vi "New Project.vi"(9 "DBSet":T1={"Server"="172.20.23.107", "DB"="HTPSDB", "PSW"="data'songyy", "User"="sa"}, 10 "UserID":string="L043460", 11 "厂区":string="清溪") -> ()   [LabVIEW 2011] (continued)
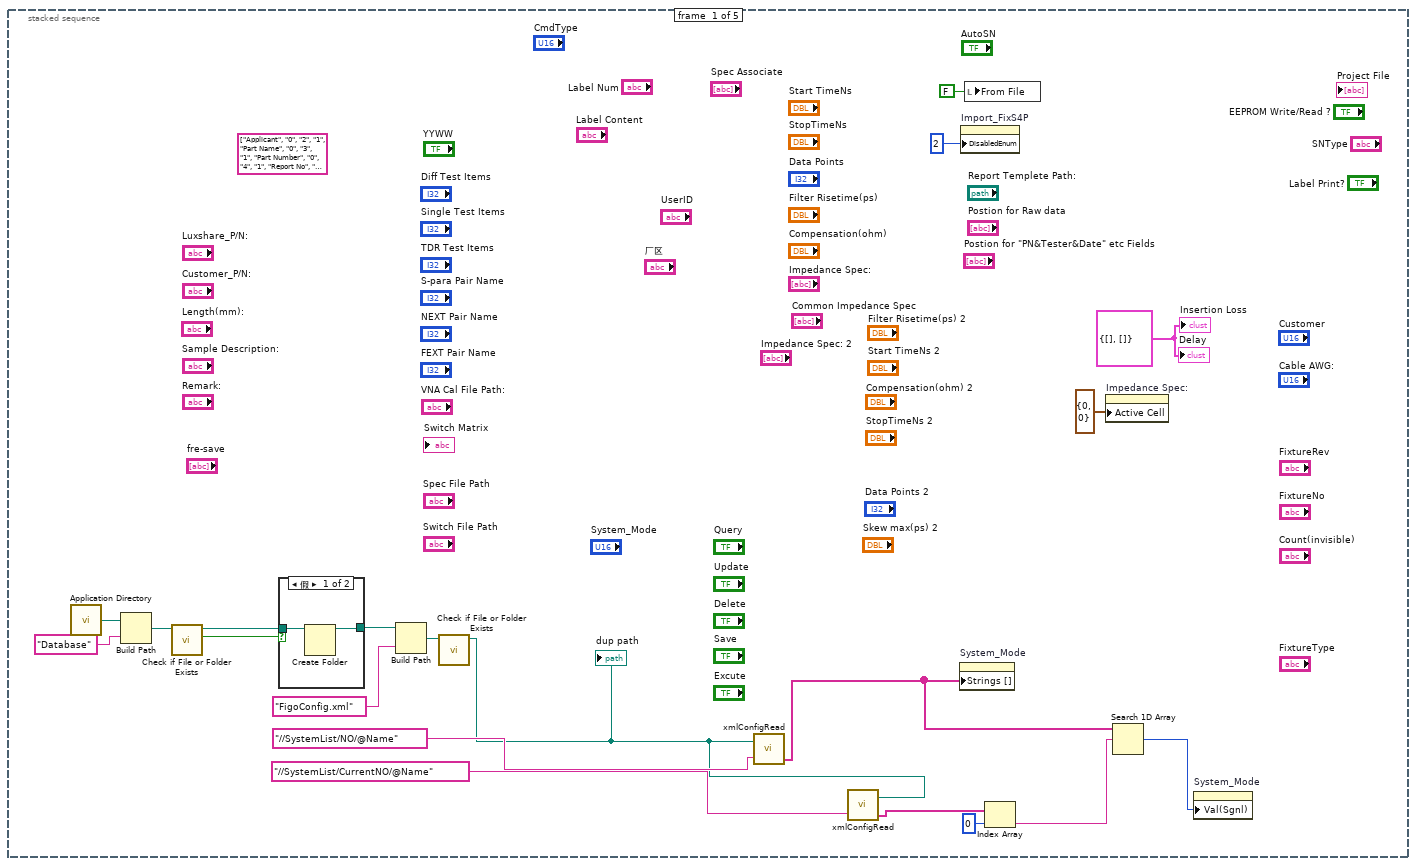
[diagram p3: hidden frame]
                          }
                          frame True {
                            n930 = local read "Luxshare_P/N:"() -> (w1140:string)
                            n931 = local read "Project File"() -> (w1139:string[])
                            n932 = local read "Local"() -> (w1138:bool)
                            n933 = case shown="真" w1138 {
                              tunnel: w1139 -> [w1145 w1157]
                              tunnel: w1140 -> [_ w1165]
                              tunnel: w1137 -> [w1141 _]
                              frame False {
                                (unwired) string[] ["LuxsharePN", "CustomerPN", "Customer", "Prjinf", "SampleDes", "AWG", "Length", "Spec", "SwitchMatrix", "EEPROMTF", "FixtureNo", "LabelTF", "LabelNum", "LabelC", "Remark", "AutoSN", "FrePoints"] ("列名")
                                # "保存至数据库"
                                n934 = call "sql-writeinfo_vproject.vi"("操作模式"=enum16{"写入数据", "更改数据"}."写入数据", "列名"=string[] ["LuxsharePN", "CustomerPN", "Customer", "Prjinf", "SampleDes", "AWG", "Length", "Spec", "SwitchMatrix", "EEPROMTF", "FixtureNo", "LabelTF", "LabelNum", "LabelC", "Remark", "AutoSN", "FrePoints", "Switch_File_Path", "Spec_File_Path", "Spec_Points", "HardWare_Mode", "Factory", "LastLog"], "DBSet"=w1141, "值"=w1145) -> ("简单报错"=w1143:string, "status"=w1144:bool)  [unwired: 14 in]
                                n935 = case shown="假" w1144 {
                                tunnel: w1143 -> [_ w1156]
                                frame False {
                                # "清空操作"
                                n936 = control-ref of="Spec Associate"() -> (w1147:refnum<vi>)
                                n937 = control-ref of="Report Templete Path:"() -> (w1150:refnum<vi>)
                                n938 = control-ref of="Data Points"() -> (w1149:refnum<vi>)
                                n939 = local read "bool"() -> (w1148:refnum<vi>[])
                                n940 = One Button Dialog(message="Save Finished!" ("消息")) -> ()  [unwired: 1 in, 1 out]
                                n941 = local read "number"() -> (w1151:refnum<vi>[])
                                n942 = local read "string"() -> (w1154:refnum<vi>[])
                                n943 = local read "chart"() -> (w1152:refnum<vi>[])
                                n944 = local read "list"() -> (w1153:refnum<vi>[])
                                n945 = call "_wmg_initAllCtrls.vi"("chart"=w1152, "number"=w1151, "list"=w1153, "string"=w1154, "bool"=w1148, "Spec _Data"=w1147, "Data Points"=w1149, "Report Templete Path:"=w1150) -> ()
                                }
                                frame True {
                                n946 = One Button Dialog(message=w1156) -> ()  [unwired: 1 in, 1 out]
                                }
                                }
                              }
                              frame True {
                                n947 = call <vilib>:"Application Directory.vi"() -> ("Application Directory"=w1164:path)
                                n948 = Concatenate Strings("Database\\" ("字符串"), w1165, ".hpj" ("字符串")) -> (w1163:string)
                                n949 = Build Path(base path=w1164, name or relative path=w1163) -> (appended path=w1160:path)
                                n950 = call <vilib>:"Check if File or Folder Exists.vi"("path"=w1160) -> ("file or folder exists?"=w1159:bool, "dup path"=w1158:path)  [unwired: 8 in, 1 out]
                                n951 = case shown="真" w1159 {
                                tunnel: w1158 -> [w1169 w1179]
                                tunnel: w1157 -> [w1168 w1178]
                                frame False {
                                # "清空操作"
                                n952 = control-ref of="Spec Associate"() -> (w1166:refnum<vi>)
                                n953 = One Button Dialog(message="Local file save Finished!" ("消息")) -> ()  [unwired: 1 in, 1 out]
                                n954 = control-ref of="Report Templete Path:"() -> (w1175:refnum<vi>)
                                n955 = control-ref of="Data Points"() -> (w1176:refnum<vi>)
                                n956 = local read "bool"() -> (w1167:refnum<vi>[])
                                n957 = Write to Binary File(file (use dialog)=w1169, data=w1168, 9:T8."big-endian, network order" ("字节顺序(0:big-endian, network order)")) -> ()  [unwired: 3 in, 3 out]
                                n958 = local read "number"() -> (w1174:refnum<vi>[])
                                n959 = local read "string"() -> (w1171:refnum<vi>[])
                                n960 = local read "chart"() -> (w1173:refnum<vi>[])
                                n961 = local read "list"() -> (w1172:refnum<vi>[])
                                n962 = call "_wmg_initAllCtrls.vi"("chart"=w1173, "number"=w1174, "list"=w1172, "string"=w1171, "bool"=w1167, "Spec _Data"=w1166, "Data Points"=w1176, "Report Templete Path:"=w1175) -> ()
                                }
                                frame True {
                                n963 = Two Button Dialog(message="该PN的文件已经存在\n是否覆盖？", 1:"取消" ("F按钮名称（“取消”）"), 2:"覆盖" ("T按钮名称（“确定”）")) -> (T button?=w1180:bool)
                                n964 = case shown="真" w1180 {
                                tunnel: w1179 -> [_ w1185]
                                tunnel: w1178 -> [_ w1184]
                                frame False {
                                }
                                frame True {
                                n965 = stacked-sequence {
                                tunnel: w1185 -> [w1188 _]
                                tunnel: w1184 -> [w1186 _]
                                frame #0 {
                                n966 = One Button Dialog(message="Coved successfully!" ("消息")) -> ()  [unwired: 1 in, 1 out]
                                n967 = Write to Binary File(file (use dialog)=w1188, data=w1186, 9:T8."big-endian, network order" ("字节顺序(0:big-endian, network order)")) -> ()  [unwired: 3 in, 3 out]
                                }
                                frame #1 {
                                # "清空操作"
                                n968 = control-ref of="Report Templete Path:"() -> (w1195:refnum<vi>)
                                n969 = control-ref of="Data Points"() -> (w1196:refnum<vi>)
                                n970 = control-ref of="Spec Associate"() -> (w1190:refnum<vi>)
                                n971 = local read "number"() -> (w1194:refnum<vi>[])
                                n972 = local read "string"() -> (w1191:refnum<vi>[])
                                n973 = local read "chart"() -> (w1193:refnum<vi>[])
                                n974 = local read "list"() -> (w1192:refnum<vi>[])
                                n975 = call "_wmg_initAllCtrls.vi"("chart"=w1193, "number"=w1194, "list"=w1192, "string"=w1191, "Spec _Data"=w1190, "Data Points"=w1196, "Report Templete Path:"=w1195) -> ()  [unwired: 1 in]
                                }
                                }
                                }
                                }
                                }
                                }
                              }
                            }
                          }
                        }
                      }
                      frame #5 {
                        n976 = property on="Update" class="Bool (严格)"("DisabledEnum"=T5."Disabled and Grayed Out" ("禁用")) -> ()  [unwired: 2 in, 2 out]
                        n977 = property on="Delete" class="Bool (严格)"("DisabledEnum"=T5."Disabled and Grayed Out" ("禁用")) -> ()  [unwired: 2 in, 2 out]
                        n978 = property on="Luxshare_P/N:" class="Str"("DisabledEnum"=T5."Disabled and Grayed Out" ("禁用")) -> ()  [unwired: 2 in, 2 out]
                        n979 = local write "Query"(FALSE ("Query")) -> ()
                        n980 = local write "Update"(FALSE ("Query")) -> ()
                        n981 = local write "Delete"(FALSE ("Query")) -> ()
                        n982 = local write "Save"(FALSE ("Query")) -> ()
                      }
                    }
                  }
                  frame #2 {
                    w1205 = u16 0 items=["", "Common", "H3C psw 10G", "H3C psw 28G"] ("CmdType")
                    # "清空数组"
                    n983 = control-ref of="Spec Associate"() -> (w1204:refnum<vi>)
                    n984 = control-ref of="Report Templete Path:"() -> (w1208:refnum<vi>)
                    n985 = control-ref of="Data Points"() -> (w1207:refnum<vi>)
                    n986 = local write "CmdType"(w1205) -> ()
                    n987 = local read "bool"() -> (w1206:refnum<vi>[])
                    n988 = local read "number"() -> (w1209:refnum<vi>[])
                    n989 = local read "string"() -> (w1212:refnum<vi>[])
                    n990 = local read "chart"() -> (w1210:refnum<vi>[])
                    n991 = local read "list"() -> (w1211:refnum<vi>[])
                    n992 = call "_wmg_initAllCtrls.vi"("chart"=w1210, "number"=w1209, "list"=w1211, "string"=w1212, "bool"=w1206, "Spec _Data"=w1204, "Data Points"=w1207, "Report Templete Path:"=w1208) -> ()
                    n993 = property on="Update" class="Bool (严格)"("DisabledEnum"=T5."Disabled and Grayed Out" ("禁用")) -> ()  [unwired: 2 in, 2 out]
                    n994 = property on="Delete" class="Bool (严格)"("DisabledEnum"=T5."Disabled and Grayed Out" ("禁用")) -> ()  [unwired: 2 in, 2 out]
                    n995 = property on="Luxshare_P/N:" class="Str"("DisabledEnum"=T5."Disabled and Grayed Out" ("禁用")) -> ()  [unwired: 2 in, 2 out]
                    n996 = local write "Query"(FALSE ("Query")) -> ()
                    n997 = local write "Update"(FALSE ("Query")) -> ()
                    n998 = local write "Delete"(FALSE ("Query")) -> ()
                    n999 = local write "Save"(FALSE ("Query")) -> ()
                  }
                }
              }
              frame 10 {
                # "delete"
                n1000 = stacked-sequence {
                  tunnel: w1220 -> [w1221 _]
                  frame #0 {
                    n1001 = local read "Local"() -> (w1222:bool)
                    n1002 = case shown="假" w1222 {
                      tunnel: w1221 -> [w1223 _]
                      frame False {
                        n1003 = local read "Luxshare_P/N:"() -> (w1232:string)
                        n1004 = property on="System_Mode" class="Ring (严格)"() -> ("RingText.Text"=w1228:string)  [unwired: 2 in, 2 out]
                        n1005 = local read "厂区"() -> (w1224:string)
                        n1006 = call "_wmg_HardModetoHardModewhereConnect.vi"("Input"=w1228, "Factory"=w1224) -> ("Output"=w1226:string)
                        n1007 = call "_wmg_PNtoPNwhereConnect.vi"("Input"=w1232) -> ("Output"=w1227:string)
                        n1008 = Concatenate Strings(w1227, w1226) -> (w1225:string)
                        n1009 = call "sql-delete.vi"("操作模式"=T9."删除数据", "DBSet"=w1223, "限定条件"=w1225) -> ("错误类型"=w1229:string, "status"=w1230:bool)  [unwired: 15 in]
                        n1010 = case shown="假" w1230 {
                          tunnel: ["数据删除成功！" ("消息") w1235] -> w1231
                          tunnel: w1229 -> [_ w1235]
                          frame False {
                          }
                          frame True {
                          }
                        }
                        n1011 = One Button Dialog(message=w1231) -> ()  [unwired: 1 in, 1 out]
                      }
                      frame True {
                        n1012 = local read "Luxshare_P/N:"() -> (w1241:string)
                        n1013 = call <vilib>:"Application Directory.vi"() -> ("Application Directory"=w1245:path)
                        n1014 = Concatenate Strings("Database\\" ("字符串"), w1241, ".hpj" ("字符串")) -> (w1244:string)
                        n1015 = Build Path(base path=w1245, name or relative path=w1244) -> (appended path=w1240:path)
                        n1016 = Delete(path (use dialog)=w1240) -> (error out=w1236:errorcluster)  [unwired: 4 in, 2 out]
                        n1017 = Unbundle(w1236) -> ("status"=w1239:bool, "source"=w1237:string)  [unwired: 1 out]
                        n1018 = case shown="假" w1239 {
                          tunnel: ["文件删除成功！" ("消息") w1247] -> w1238
                          tunnel: w1237 -> [_ w1247]
                          frame False {
                          }
                          frame True {
                          }
                        }
                        n1019 = One Button Dialog(message=w1238) -> ()  [unwired: 1 in, 1 out]
                      }
                    }
                  }
                  frame #1 {
                    w1249 = u16 0 items=["", "Common", "H3C psw 10G", "H3C psw 28G"] ("CmdType")
                    # "清空数组"
                    n1020 = control-ref of="Spec Associate"() -> (w1248:refnum<vi>)
                    n1021 = control-ref of="Report Templete Path:"() -> (w1259:refnum<vi>)
                    n1022 = control-ref of="Data Points"() -> (w1258:refnum<vi>)
                    n1023 = local write "CmdType"(w1249) -> ()
                    n1024 = local read "bool"() -> (w1250:refnum<vi>[])
                    n1025 = local read "number"() -> (w1260:refnum<vi>[])
                    n1026 = local read "string"() -> (w1263:refnum<vi>[])
                    n1027 = local read "chart"() -> (w1261:refnum<vi>[])
                    n1028 = local read "list"() -> (w1262:refnum<vi>[])
                    n1029 = call "_wmg_initAllCtrls.vi"("chart"=w1261, "number"=w1260, "list"=w1262, "string"=w1263, "bool"=w1250, "Spec _Data"=w1248, "Data Points"=w1258, "Report Templete Path:"=w1259) -> ()
                    n1030 = property on="Update" class="Bool (严格)"("DisabledEnum"=T5."Disabled and Grayed Out" ("禁用")) -> ()  [unwired: 2 in, 2 out]
                    n1031 = property on="Delete" class="Bool (严格)"("DisabledEnum"=T5."Disabled and Grayed Out" ("禁用")) -> ()  [unwired: 2 in, 2 out]
                    n1032 = property on="Luxshare_P/N:" class="Str"("DisabledEnum"=T5."Disabled and Grayed Out" ("禁用")) -> ()  [unwired: 2 in, 2 out]
                    n1033 = local write "Query"(FALSE ("Query")) -> ()
                    n1034 = local write "Update"(FALSE ("Query")) -> ()
                    n1035 = local write "Delete"(FALSE ("Query")) -> ()
                    n1036 = local write "Save"(FALSE ("Query")) -> ()
                  }
                }
              }
              frame 1 {
                # "save"
                n1037 = stacked-sequence {
                  tunnel: w1264 -> [_ _ _ _ w1446 _]
                  frame #0 {
                    w1291 = "@"
                    w1292 = "\r\n"
                    w1302 = "%s" ("格式字符串")
                    n1038 = local read "Impedance Spec:"() -> (w1304:string[][])
                    n1039 = local read "2X Thru String"() -> (w1288:string)
                    n1040 = property on="Delay(ns)" class="DigNum (严格)"() -> ("NumText.Text"=w1286:string)  [unwired: 2 in, 2 out]
                    n1041 = property on="Skew max(ps)" class="DigNum (严格)"() -> ("NumText.Text"=w1287:string)  [unwired: 2 in, 2 out]
                    n1042 = property on="Filter Risetime(ps)" class="DigNum (严格)"() -> ("NumText.Text"=w1282:string)  [unwired: 2 in, 2 out]
                    n1043 = property on="Start TimeNs" class="DigNum (严格)"() -> ("NumText.Text"=w1285:string)  [unwired: 2 in, 2 out]
                    n1044 = property on="StopTimeNs" class="DigNum (严格)"() -> ("NumText.Text"=w1284:string)  [unwired: 2 in, 2 out]
                    n1045 = property on="Data Points" class="DigNum (严格)"() -> ("NumText.Text"=w1283:string)  [unwired: 2 in, 2 out]
                    n1046 = property on="Compensation(ohm)" class="DigNum (严格)"() -> ("NumText.Text"=w1281:string)  [unwired: 2 in, 2 out]
                    n1047 = Boolean To (0,1)(Boolean="Impedance Filter") -> (0, 1=w1307:i16)
                    n1048 = Number To Decimal String(number=w1307) -> (decimal integer string=w1305:string)  [unwired: 1 in]
                    n1049 = call "impedance spec.vi"("Impedance Spec:"=w1304) -> ("Impedance spec string"=w1303:string)  [unwired: 10 in]
                    n1050 = call <vilib>:"Trim Whitespace.vi"("string"=w1288) -> ("trimmed string"=w1280:string)  [unwired: 1 in]
                    n1051 = Build Array(w1285, w1284, w1283, w1282, w1281, w1305, w1303, w1286, w1287, w1280) -> (→"TDR Setting":string[])
                    n1052 = local read "Impedance Spec: 2"() -> (w1270:string[][])
                    n1053 = local read "Report Templete Path:"() -> (w1289:path)
                    n1054 = property on="Delay(ns)" class="DigNum (严格)"() -> ("NumText.Text"=w1268:string)  [unwired: 2 in, 2 out]
                    n1055 = property on="Skew max(ps) 2" class="DigNum (严格)"() -> ("NumText.Text"=w1267:string)  [unwired: 2 in, 2 out]
                    n1056 = local read "2X Thru String"() -> (w1277:string)
                    n1057 = property on="Postion for Raw data" class="Tbl (严格)"() -> ("Value"=w1301:string[][])  [unwired: 2 in, 2 out]
                    n1058 = property on="Start TimeNs 2" class="DigNum (严格)"() -> ("NumText.Text"=w1276:string)  [unwired: 2 in, 2 out]
                    n1059 = property on="StopTimeNs 2" class="DigNum (严格)"() -> ("NumText.Text"=w1275:string)  [unwired: 2 in, 2 out]
                    n1060 = property on="Data Points 2" class="DigNum (严格)"() -> ("NumText.Text"=w1274:string)  [unwired: 2 in, 2 out]
                    n1061 = property on="Filter Risetime(ps) 2" class="DigNum (严格)"() -> ("NumText.Text"=w1273:string)  [unwired: 2 in, 2 out]
                    n1062 = property on="Compensation(ohm) 2" class="DigNum (严格)"() -> ("NumText.Text"=w1272:string)  [unwired: 2 in, 2 out]
                    n1063 = property on="Postion for \"PN&Tester&Date\" etc Fields" class="Tbl (严格)"() -> ("Value"=w1300:string[][])  [unwired: 2 in, 2 out]
                    n1064 = Boolean To (0,1)(Boolean="Impedance Filter 2") -> (0, 1=w1278:i16)
                    n1065 = Array To Spreadsheet String(array=w1301, 3:w1302) -> (spreadsheet string=w1297:string)  [unwired: 1 in]
                    n1066 = Array To Spreadsheet String(array=w1300, 3:w1302) -> (spreadsheet string=w1295:string)  [unwired: 1 in]
                    n1067 = Number To Decimal String(number=w1278) -> (decimal integer string=w1271:string)  [unwired: 1 in]
                    n1068 = call "impedance spec.vi"("Impedance Spec:"=w1270) -> ("Impedance spec string"=w1269:string)  [unwired: 10 in]
                    n1069 = call <vilib>:"Trim Whitespace.vi"("string"=w1277) -> ("trimmed string"=w1266:string)  [unwired: 1 in]
                    n1070 = Path To String(path=w1289) -> (string=w1290:string)
                    n1071 = Search and Replace String(replace all?=TRUE ("替换全部？(F)"), input string=w1297, search string=w1292, replace string=w1291) -> (result string=w1294:string)  [unwired: 4 in, 3 out]
                    n1072 = Search and Replace String(replace all?=TRUE ("替换全部？(F)"), input string=w1295, search string=w1292, replace string=w1291) -> (result string=w1293:string)  [unwired: 4 in, 3 out]
                    n1073 = Build Array(w1276, w1275, w1274, w1273, w1272, w1271, w1269, w1268, w1267, w1266) -> (→"TDR Setting2":string[])
                    n1074 = Build Array(w1290, w1294, w1293) -> (→"Report Config":string[])
                  }
                  frame #1 {
                    n1075 = local read "Common Impedance Spec"() -> (w1312:string[][])
                    n1076 = property on="S-para Pair Name" class="LstBox (严格)"() -> ("Item Names"=w1344:string[], "Item Symbols"=w1343:i32[])  [unwired: 2 in, 2 out]
                    n1077 = property on="NEXT Pair Name" class="LstBox (严格)"() -> ("Item Names"=w1342:string[], "Item Symbols"=w1341:i32[])  [unwired: 2 in, 2 out]
                    n1078 = property on="FEXT Pair Name" class="LstBox (严格)"() -> ("Item Names"=w1340:string[], "Item Symbols"=w1339:i32[])  [unwired: 2 in, 2 out]
                    n1079 = property on="Single Test Items" class="LstBox (严格)"() -> ("Item Names"=w1346:string[], "Item Symbols"=w1345:i32[])  [unwired: 2 in, 2 out]
                    n1080 = property on="Diff Test Items" class="LstBox (严格)"() -> ("Item Names"=w1348:string[], "Item Symbols"=w1347:i32[])  [unwired: 2 in, 2 out]
                    n1081 = property on="TDR Test Items" class="LstBox (严格)"() -> ("Item Names"=w1324:string[], "Item Symbols"=w1323:i32[])  [unwired: 2 in, 2 out]
                    n1082 = call "Selected items.vi"("Item Syms"=w1343, "Item name"=w1344) -> ("Selected tem"=w1338:string[])  [unwired: 7 in, 2 out]
                    n1083 = call "Selected items.vi"("Item Syms"=w1341, "Item name"=w1342) -> ("Selected tem"=w1337:string[])  [unwired: 7 in, 2 out]
                    n1084 = call "Selected items.vi"("Item Syms"=w1339, "Item name"=w1340) -> ("Selected tem"=w1336:string[])  [unwired: 7 in, 2 out]
                    n1085 = call "Selected items.vi"("Item Syms"=w1347, "Item name"=w1348) -> ("Selected tem"=w1335:string[])  [unwired: 7 in, 2 out]
                    n1086 = call "Selected items.vi"("Item Syms"=w1345, "Item name"=w1346) -> ("Selected tem"=w1334:string[])  [unwired: 7 in, 2 out]
                    n1087 = call "Selected items.vi"("Item Syms"=w1323, "Item name"=w1324) -> ("Selected tem"=w1322:string[])  [unwired: 7 in, 2 out]
                    n1088 = call "impedance spec.vi"("Impedance Spec:"=w1312) -> ("Impedance spec string"=w1311:string)  [unwired: 10 in]
                    n1089 = local read "VNA Cal File Path:"() -> (w1319:string)
                    n1090 = Build Array(w1311) -> (w1310:string[])
                    n1091 = local read "Report Config"() -> (w1320:string[])
                    n1092 = local read "Cancel Dem2X?"() -> (w1317:bool)
                    n1093 = local read "TDR Setting2"() -> (w1318:string[])
                    n1094 = local read "TDR Setting"() -> (w1321:string[])
                    n1095 = Build Array(w1319) -> (w1333:string[])
                    n1096 = Number To Decimal String(number="ILD Spec") -> (decimal integer string=w1326:string)  [unwired: 1 in]
                    n1097 = Build Array(w1326) -> (w1325:string[])
                    n1098 = Select(t="TRUE", s=w1317, f="FALSE") -> (s? t:f=w1314:string)
                    n1099 = Build Array(w1314) -> (w1313:string[])
                    n1100 = Build Array(w1338, w1337, w1336, w1335, w1334, w1322, string[] ["占位符"], w1333, w1320, w1325, w1321, w1318, w1313, w1310) -> (w1332:string[][])
                    n1101 = Transpose 2D Array(2D array=w1332) -> (transposed array=w1331:string[][])
                    n1102 = Array To Spreadsheet String(delimiter (Tab)="#" ("分隔符(Tab)"), array=w1331, 3:"%s" ("格式字符串")) -> (spreadsheet string=→"Project Information":string)
                  }
                  frame #2 {
                    n1103 = local read "VNA Cal File Path:"() -> (w1368:string)
                    n1104 = property on="Diff Test Items" class="LstBox (严格)"() -> ("Item Symbols"=w1365:i32[])  [unwired: 2 in, 2 out]
                    n1105 = property on="Single Test Items" class="LstBox (严格)"() -> ("Item Symbols"=w1364:i32[])  [unwired: 2 in, 2 out]
                    n1106 = property on="TDR Test Items" class="LstBox (严格)"() -> ("Item Symbols"=w1363:i32[])  [unwired: 2 in, 2 out]
                    n1107 = property on="S-para Pair Name" class="LstBox (严格)"() -> ("Item Symbols"=w1362:i32[])  [unwired: 2 in, 2 out]
                    n1108 = property on="NEXT Pair Name" class="LstBox (严格)"() -> ("Item Symbols"=w1361:i32[])  [unwired: 2 in, 2 out]
                    n1109 = property on="FEXT Pair Name" class="LstBox (严格)"() -> ("Item Symbols"=w1357:i32[])  [unwired: 2 in, 2 out]
                    n1110 = local read "Luxshare_P/N:"() -> (w1355:string)
                    n1111 = local read "Length(mm):"() -> (w1369:string)
                    n1112 = String Length(string=w1355) -> (length=w1356:i32)
                    n1113 = Empty String/Path?(string/path=w1368) -> (empty?=w1366:bool)
                    n1114 = Empty String/Path?(string/path=w1369) -> (empty?=w1367:bool)
                    n1115 = Build Array(w1365, w1364, w1363, w1362, w1361, w1357) -> (w1360:i32[][])
                    n1116 = Not(x=w1367) -> (.not. x?=w1359:bool)
                    n1117 = Not(x=w1366) -> (.not. x?=w1358:bool)
                    n1118 = Greater Than 0?(x=w1356) -> (x > 0?=w1354:bool)
                    n1119 = local read "Spec Associate"() -> (w1349:string[][])
                    n1120 = call "_wmg_whetherItemsEmpty.vi"("Input"=w1360) -> ("bool"=w1370:bool)
                    n1121 = Compound Arithmetic op=AND(w1354, w1359, w1358, w1370) -> (→"save?":bool)
                    n1122 = Array To Spreadsheet String(delimiter (Tab)="#" ("分隔符(Tab)"), array=w1349, 3:"%s" ("格式字符串")) -> (spreadsheet string=w1352:string)
                    n1123 = local write "Spec String"(w1352) -> ()
                  }
                  frame #3 {
                    n1124 = local read "Local"() -> (w1371:bool)
                    n1125 = case shown="真" w1371 {
                      frame False {
                        # "16"
                        # "15"
                        # "14"
                        # "13"
                        # "11"
                        # "10"
                        # "9"
                        # "8"
                        # "7"
                        # "6"
                        # "5"
                        # "4"
                        # "3"
                        # "2"
                        # "1"
                        n1126 = local read "Label Print?"() -> (w1383:bool)
                        n1127 = local read "UserID"() -> (w1375:string)
                        n1128 = local read "fre-save"() -> (w1390:string[])
                        n1129 = Format Date/Time String(time format string (%c)="%Y-%m-%d : %H:%M" ("时间格式字符串(%c)")) -> (date/time string=w1372:string)  [unwired: 2 in]
                        n1130 = Boolean To (0,1)(Boolean=w1383) -> (0, 1=w1408:i16)
                        n1131 = local read "EEPROM Write/Read ?"() -> (w1384:bool)
                        n1132 = local read "Sample Description:"() -> (w1404:string)
                        n1133 = local read "Project Information"() -> (w1405:string)
                        n1134 = Array To Spreadsheet String(delimiter (Tab)="," ("分隔符(Tab)"), array=w1390, 3:"" ("格式字符串")) -> (spreadsheet string=w1387:string)
                        n1135 = Number To Decimal String(number=w1408) -> (decimal integer string=w1398:string)  [unwired: 1 in]
                        n1136 = local read "Customer_P/N:"() -> (w1407:string)
                        n1137 = local read "Switch Matrix"() -> (w1400:string)
                        n1138 = local read "Label Content"() -> (w1397:string)
                        n1139 = local read "Length(mm):"() -> (w1402:string)
                        n1140 = local read "Spec String"() -> (w1401:string)
                        n1141 = call <vilib>:"Trim Whitespace.vi"("string"=w1387) -> ("trimmed string"=w1386:string)  [unwired: 1 in]
                        n1142 = Concatenate Strings(w1375, " saved@" ("字符串"), w1372) -> (w1374:string)
                        n1143 = property on="Customer" class="Ring (严格)"() -> ("RingText.Text"=w1406:string)  [unwired: 2 in, 2 out]
                        n1144 = property on="Cable AWG:" class="Ring (严格)"() -> ("RingText.Text"=w1403:string)  [unwired: 2 in, 2 out]
                        n1145 = local read "FixtureNo"() -> (w1395:string)
                        n1146 = local read "Label Num"() -> (w1410:string)
                        n1147 = local read "Remark:"() -> (w1396:string)
                        n1148 = local read "厂区"() -> (w1377:string)
                        n1149 = local read "Switch File Path"() -> (w1382:string)
                        n1150 = Boolean To (0,1)(Boolean=w1384) -> (0, 1=w1409:i16)
                        n1151 = local read "AutoSN"() -> (w1392:bool)
                        n1152 = Number To Decimal String(number=w1409) -> (decimal integer string=w1399:string)  [unwired: 1 in]
                        n1153 = Boolean To (0,1)(Boolean=w1392) -> (0, 1=w1393:i16)
                        n1154 = local read "Spec File Path"() -> (w1381:string)
                        n1155 = Number To Decimal String(number=w1393) -> (decimal integer string=w1391:string)  [unwired: 1 in]
                        n1156 = local read "Luxshare_P/N:"() -> (w1394:string)
                        n1157 = local read "Spec Points"() -> (w1380:dbl)
                        n1158 = property on="System_Mode" class="Ring (严格)"() -> ("RingText.Text"=w1378:string)  [unwired: 2 in, 2 out]
                        n1159 = Number To Decimal String(number=w1380) -> (decimal integer string=w1379:string)  [unwired: 1 in]
                        n1160 = Build Array(w1394, w1407, w1406, w1405, w1404, w1403, w1402, w1401, w1400, w1399, w1395, w1398, w1410, w1397, w1396, w1391, w1386, w1382, w1381, w1379, w1378, w1377, w1374) -> (w1385:string[])
                        n1161 = local write "Project File"(w1385) -> ()
                      }
                      frame True {
                        # "11"
                        # "10"
                        # "9"
                        # "8"
                        # "7"
                        # "6"
                        # "5"
                        # "4"
                        # "3"
                        # "2"
                        # "1"
                        n1162 = local read "Label Print?"() -> (w1416:bool)
                        n1163 = local read "fre-save"() -> (w1424:string[])
                        n1164 = Boolean To (0,1)(Boolean=w1416) -> (0, 1=w1443:i16)
                        n1165 = local read "EEPROM Write/Read ?"() -> (w1418:bool)
                        n1166 = property on="CmdType" class="Ring (严格)"() -> ("RingText.Text"=w1415:string)  [unwired: 2 in, 2 out]
                        n1167 = local read "Sample Description:"() -> (w1439:string)
                        n1168 = local read "Project Information"() -> (w1440:string)
                        n1169 = Array To Spreadsheet String(delimiter (Tab)="," ("分隔符(Tab)"), array=w1424, 3:"" ("格式字符串")) -> (spreadsheet string=w1421:string)
                        n1170 = local read "SNType"() -> (w1417:string)
                        n1171 = Number To Decimal String(number=w1443) -> (decimal integer string=w1433:string)  [unwired: 1 in]
                        n1172 = local read "Customer_P/N:"() -> (w1442:string)
                        n1173 = local read "Switch Matrix"() -> (w1435:string)
                        n1174 = local read "Label Content"() -> (w1432:string)
                        n1175 = local read "Length(mm):"() -> (w1437:string)
                        n1176 = local read "Spec String"() -> (w1436:string)
                        n1177 = call <vilib>:"Trim Whitespace.vi"("string"=w1421) -> ("trimmed string"=w1420:string)  [unwired: 1 in]
                        n1178 = property on="Customer" class="Ring (严格)"() -> ("RingText.Text"=w1441:string)  [unwired: 2 in, 2 out]
                        n1179 = property on="Cable AWG:" class="Ring (严格)"() -> ("RingText.Text"=w1438:string)  [unwired: 2 in, 2 out]
                        n1180 = local read "FixtureNo"() -> (w1430:string)
                        n1181 = local read "Label Num"() -> (w1445:string)
                        n1182 = local read "Remark:"() -> (w1431:string)
                        n1183 = call <vilib>:"Trim Whitespace.vi"("string"=w1415) -> ("trimmed string"=w1428:string)  [unwired: 1 in]
                        n1184 = local read "Switch File Path"() -> (w1414:string)
                        n1185 = Boolean To (0,1)(Boolean=w1418) -> (0, 1=w1444:i16)
                        n1186 = local read "AutoSN"() -> (w1426:bool)
                        n1187 = Number To Decimal String(number=w1444) -> (decimal integer string=w1434:string)  [unwired: 1 in]
                        n1188 = Boolean To (0,1)(Boolean=w1426) -> (0, 1=w1427:i16)
                        n1189 = Number To Decimal String(number=w1427) -> (decimal integer string=w1425:string)  [unwired: 1 in]
                        n1190 = local read "Luxshare_P/N:"() -> (w1429:string)
                        n1191 = local read "Spec File Path"() -> (w1413:string)
                        n1192 = local read "Spec Points"() -> (w1412:dbl)
                        n1193 = Number To Decimal String(number=w1412) -> (decimal integer string=w1411:string)  [unwired: 1 in]
                        n1194 = Build Array(w1429, w1442, w1441, w1440, w1439, w1438, w1437, w1436, w1435, w1434, w1428, w1417, w1430, w1433, w1445, w1432, w1431, w1425, w1420, w1414, w1413, w1411) -> (w1419:string[])
                        n1195 = local write "Project File"(w1419) -> ()
                      }
                    }
                  }
                  frame #4 {
                    n1196 = local read "save?"() -> (w1447:bool)
                    n1197 = case shown="真" w1447 {
                      tunnel: w1446 -> [_ w1449]
                      frame False {
                        n1198 = One Button Dialog(message="保存信息不完整" ("消息")) -> ()  [unwired: 1 in, 1 out]
                      }
                      frame True {
                        n1199 = local read "Luxshare_P/N:"() -> (w1451:string)
                        n1200 = local read "Project File"() -> (w1450:string[])
                        n1201 = case shown="真" "Local" {
                          tunnel: w1450 -> [w1457 w1469]
                          tunnel: w1451 -> [_ w1477]
                          tunnel: w1449 -> [w1453 _]
                          frame False {
                            # "保存至数据库"
                            n1202 = call "sql-writeinfo_vproject.vi"("操作模式"=enum16{"写入数据", "更改数据"}."写入数据", "列名"=string[] ["LuxsharePN", "CustomerPN", "Customer", "Prjinf", "SampleDes", "AWG", "Length", "Spec", "SwitchMatrix", "EEPROMTF", "FixtureNo", "LabelTF", "LabelNum", "LabelC", "Remark", "AutoSN", "FrePoints", "Switch_File_Path", "Spec_File_Path", "Spec_Points", "HardWare_Mode", "Factory", "LastLog"], "DBSet"=w1453, "值"=w1457) -> ("简单报错"=w1455:string, "status"=w1456:bool)  [unwired: 14 in]
                            n1203 = case shown="假" w1456 {
                              tunnel: w1455 -> [_ w1468]
                              frame False {
                                # "清空操作"
                                n1204 = control-ref of="Spec Associate"() -> (w1459:refnum<vi>)
                                n1205 = control-ref of="Report Templete Path:"() -> (w1462:refnum<vi>)
                                n1206 = control-ref of="Data Points"() -> (w1461:refnum<vi>)
                                n1207 = local read "bool"() -> (w1460:refnum<vi>[])
                                n1208 = One Button Dialog(message="Save Finished!" ("消息")) -> ()  [unwired: 1 in, 1 out]
                                n1209 = local read "number"() -> (w1463:refnum<vi>[])
                                n1210 = local read "string"() -> (w1466:refnum<vi>[])
                                n1211 = local read "chart"() -> (w1464:refnum<vi>[])
                                n1212 = local read "list"() -> (w1465:refnum<vi>[])
                                n1213 = call "_wmg_initAllCtrls.vi"("chart"=w1464, "number"=w1463, "list"=w1465, "string"=w1466, "bool"=w1460, "Spec _Data"=w1459, "Data Points"=w1461, "Report Templete Path:"=w1462) -> ()
                              }
                              frame True {
                                n1214 = One Button Dialog(message=w1468) -> ()  [unwired: 1 in, 1 out]
                              }
                            }
                          }
                          frame True {
                            n1215 = call <vilib>:"Application Directory.vi"() -> ("Application Directory"=w1476:path)
                            n1216 = Concatenate Strings("Database\\" ("字符串"), w1477, ".hpj" ("字符串")) -> (w1475:string)
                            n1217 = Build Path(base path=w1476, name or relative path=w1475) -> (appended path=w1472:path)
                            n1218 = call <vilib>:"Check if File or Folder Exists.vi"("path"=w1472) -> ("file or folder exists?"=w1471:bool, "dup path"=w1470:path)  [unwired: 8 in, 1 out]
                            n1219 = case shown="假" w1471 {
                              tunnel: w1470 -> [w1481 w1491]
                              tunnel: w1469 -> [w1480 w1490]
                              frame False {
                                # "清空操作"
                                n1220 = control-ref of="Spec Associate"() -> (w1478:refnum<vi>)
                                n1221 = One Button Dialog(message="Local file save Finished!" ("消息")) -> ()  [unwired: 1 in, 1 out]
                                n1222 = control-ref of="Report Templete Path:"() -> (w1487:refnum<vi>)
                                n1223 = control-ref of="Data Points"() -> (w1488:refnum<vi>)
                                n1224 = local read "bool"() -> (w1479:refnum<vi>[])
                                n1225 = Write to Binary File(file (use dialog)=w1481, data=w1480, 9:T8."big-endian, network order" ("字节顺序(0:big-endian, network order)")) -> ()  [unwired: 3 in, 3 out]
                                n1226 = local read "number"() -> (w1486:refnum<vi>[])
                                n1227 = local read "string"() -> (w1483:refnum<vi>[])
                                n1228 = local read "chart"() -> (w1485:refnum<vi>[])
                                n1229 = local read "list"() -> (w1484:refnum<vi>[])
                                n1230 = call "_wmg_initAllCtrls.vi"("chart"=w1485, "number"=w1486, "list"=w1484, "string"=w1483, "bool"=w1479, "Spec _Data"=w1478, "Data Points"=w1488, "Report Templete Path:"=w1487) -> ()
                              }
                              frame True {
                                n1231 = Two Button Dialog(message="该PN的文件已经存在\n是否覆盖？", 1:"取消" ("F按钮名称（“取消”）"), 2:"覆盖" ("T按钮名称（“确定”）")) -> (T button?=w1492:bool)
                                n1232 = case shown="真" w1492 {
                                tunnel: w1491 -> [_ w1497]
                                tunnel: w1490 -> [_ w1496]
                                frame False {
                                }
                                frame True {
                                n1233 = stacked-sequence {
                                tunnel: w1497 -> [w1500 _]
                                tunnel: w1496 -> [w1498 _]
                                frame #0 {
                                n1234 = One Button Dialog(message="Coved successfully!" ("消息")) -> ()  [unwired: 1 in, 1 out]
                                n1235 = Write to Binary File(file (use dialog)=w1500, data=w1498, 9:T8."big-endian, network order" ("字节顺序(0:big-endian, network order)")) -> ()  [unwired: 3 in, 3 out]
                                }
                                frame #1 {
                                # "清空操作"
                                n1236 = control-ref of="Report Templete Path:"() -> (w1507:refnum<vi>)
                                n1237 = control-ref of="Data Points"() -> (w1508:refnum<vi>)
                                n1238 = control-ref of="Spec Associate"() -> (w1502:refnum<vi>)
                                n1239 = local read "number"() -> (w1506:refnum<vi>[])
                                n1240 = local read "string"() -> (w1503:refnum<vi>[])
                                n1241 = local read "chart"() -> (w1505:refnum<vi>[])
                                n1242 = local read "list"() -> (w1504:refnum<vi>[])
                                n1243 = call "_wmg_initAllCtrls.vi"("chart"=w1505, "number"=w1506, "list"=w1504, "string"=w1503, "Spec _Data"=w1502, "Data Points"=w1508, "Report Templete Path:"=w1507) -> ()  [unwired: 1 in]
                                }
                                }
                                }
                                }
                              }
                            }
                          }
                        }
                      }
                    }
                  }
                  frame #5 {
                    w1509 = u16 0 items=["", "Common", "H3C psw 10G", "H3C psw 28G"] ("CmdType")
                    n1244 = property on="Update" class="Bool (严格)"("DisabledEnum"=T5."Disabled and Grayed Out" ("禁用")) -> ()  [unwired: 2 in, 2 out]
                    n1245 = property on="Delete" class="Bool (严格)"("DisabledEnum"=T5."Disabled and Grayed Out" ("禁用")) -> ()  [unwired: 2 in, 2 out]
                    n1246 = property on="Luxshare_P/N:" class="Str"("DisabledEnum"=T5."Disabled and Grayed Out" ("禁用")) -> ()  [unwired: 2 in, 2 out]
                    n1247 = local write "CmdType"(w1509) -> ()
                    n1248 = local write "Query"(FALSE ("Query")) -> ()
                    n1249 = local write "Update"(FALSE ("Query")) -> ()
                    n1250 = local write "Delete"(FALSE ("Query")) -> ()
                    n1251 = local write "Save"(FALSE ("Query")) -> ()
                  }
                }
              }
            }
          }
          event "System_Mode": Value Change {
            w1521 = "@NameVar@" ("搜索字符串")
            n1252 = event-data() -> ("NewVal"=w1530:u16)  [unwired: 1 in, 4 out]
            n1253 = property on="System_Mode" class="Ring (严格)"() -> ("Strings []"=w1531:string[])  [unwired: 2 in, 2 out]
            n1254 = local read "dup path"() -> (w1524:path)
            n1255 = Index Array(array=w1531, index=w1530) -> (element=w1517:string)
            n1256 = Search and Replace String(input string="//SystemList/NO[@Name='@NameVar@']/@Switch" ("XPath expression"), search string=w1521, replace string=w1517) -> (result string=w1528:string)  [unwired: 5 in, 3 out]
            n1257 = call "xmlConfigRead.vi"("path to XML document"=w1524, "XPath expression"=w1528) -> ("OutParaArray"=w1527:string[])  [unwired: 2 out]
            n1258 = Index Array(array=w1527, index=0 ("索引")) -> (element=→"开关型号":string)
            n1259 = Search and Replace String(input string="//SystemList/NO[@Name='@NameVar@']/@Equipment" ("XPath expression"), search string=w1521, replace string=w1517) -> (result string=w1523:string)  [unwired: 5 in, 3 out]
            n1260 = call "xmlConfigRead.vi"("path to XML document"=w1524, "XPath expression"=w1523) -> ("OutParaArray"=w1520:string[])  [unwired: 2 out]
            n1261 = Index Array(array=w1520, index=0 ("索引")) -> (element=→"仪器型号":string)
          }
          event Panel Close {
            n1262 = event-data() -> ()  [unwired: 1 in, 3 out]
          }
          event "Default": Value Change {
            n1263 = event-data() -> ()  [unwired: 1 in, 5 out]
            n1264 = case shown="\"Default\", 默认" "Default" {
              frame "Default", Default {
                w1534 = 0 ("Diff Test Items")
                w1540 = 37
                n1265 = local read "Inf"() -> (w1559:string[][])
                n1266 = Index Array(array=w1559, index (col) #1=0 ("禁用的索引 (列)"), index (col) #2=1 ("索引 (列)"), index (col) #3=2 ("索引 (列)"), index (col) #4=3 ("索引 (列)"), index (col) #5=4 ("索引 (列)"), index (col) #6=5 ("索引 (列)")) -> (element #1=w1553:string[], element #2=w1552:string[], element #3=w1551:string[], element #4=w1550:string[], element #5=w1549:string[], element #6=w1543:string[])  [unwired: 6 in]
                n1267 = call "Delete empty element from array.vi"("Array In"=w1543) -> ("Array out"=w1535:string[])  [unwired: 26 in]
                n1268 = call "Delete empty element from array.vi"("Array In"=w1553) -> ("Array out"=w1544:string[])  [unwired: 26 in]
                n1269 = call "Delete empty element from array.vi"("Array In"=w1549) -> ("Array out"=w1536:string[])  [unwired: 26 in]
                n1270 = call "Delete empty element from array.vi"("Array In"=w1552) -> ("Array out"=w1545:string[])  [unwired: 26 in]
                n1271 = call "Delete empty element from array.vi"("Array In"=w1551) -> ("Array out"=w1538:string[])  [unwired: 26 in]
                n1272 = call "Delete empty element from array.vi"("Array In"=w1550) -> ("Array out"=w1537:string[])  [unwired: 26 in]
                n1273 = Array Size(array=w1544) -> (size(s)=w1566:i32)
                n1274 = Array Size(array=w1545) -> (size(s)=w1560:i32)
                n1275 = Array Size(array=w1538) -> (size(s)=w1539:i32)
                n1276 = Array Size(array=w1537) -> (size(s)=w1546:i32)
                n1277 = Array Size(array=w1536) -> (size(s)=w1563:i32)
                n1278 = Array Size(array=w1535) -> (size(s)=w1547:i32)
                n1279 = Initialize Array(w1540, w1566) -> (w1565:i32[])
                n1280 = Initialize Array(w1540, w1560) -> (w1561:i32[])
                n1281 = Initialize Array(w1540, w1546) -> (w1564:i32[])
                n1282 = Initialize Array(w1540, w1539) -> (w1541:i32[])
                n1283 = Initialize Array(w1540, w1563) -> (w1562:i32[])
                n1284 = Initialize Array(w1540, w1547) -> (w1548:i32[])
                n1285 = property on="Diff Test Items" class="LstBox (严格)"("Item Names"=w1544, "Item Symbols"=w1565) -> ()  [unwired: 2 in, 2 out]
                n1286 = property on="Single Test Items" class="LstBox (严格)"("Item Names"=w1545, "Item Symbols"=w1561) -> ()  [unwired: 2 in, 2 out]
                n1287 = property on="TDR Test Items" class="LstBox (严格)"("Item Names"=w1538, "Item Symbols"=w1541) -> ()  [unwired: 2 in, 2 out]
                n1288 = property on="S-para Pair Name" class="LstBox (严格)"("Item Names"=w1537, "Item Symbols"=w1564) -> ()  [unwired: 2 in, 2 out]
                n1289 = property on="NEXT Pair Name" class="LstBox (严格)"("Item Names"=w1536, "Item Symbols"=w1562) -> ()  [unwired: 2 in, 2 out]
                n1290 = property on="FEXT Pair Name" class="LstBox (严格)"("Item Names"=w1535, "Item Symbols"=w1548) -> ()  [unwired: 2 in, 2 out]
                n1291 = property on="Diff Test Items" class="LstBox (严格)"("Value"=w1534, "Top Row"=w1534) -> ()  [unwired: 2 in, 2 out]
                n1292 = property on="Single Test Items" class="LstBox (严格)"("Value"=w1534, "Top Row"=w1534) -> ()  [unwired: 2 in, 2 out]
                n1293 = property on="TDR Test Items" class="LstBox (严格)"("Value"=w1534, "Top Row"=w1534) -> ()  [unwired: 2 in, 2 out]
                n1294 = property on="S-para Pair Name" class="LstBox (严格)"("Value"=w1534, "Top Row"=w1534) -> ()  [unwired: 2 in, 2 out]
                n1295 = property on="NEXT Pair Name" class="LstBox (严格)"("Value"=w1534, "Top Row"=w1534) -> ()  [unwired: 2 in, 2 out]
                n1296 = property on="FEXT Pair Name" class="LstBox (严格)"("Value"=w1534, "Top Row"=w1534) -> ()  [unwired: 2 in, 2 out]
              }
              frame "Quick" {
                w1567 = 0 ("Diff Test Items")
                w1571 = 38
                n1297 = local read "Inf"() -> (w1589:string[][])
                n1298 = Index Array(array=w1589, index (col) #1=0 ("禁用的索引 (列)"), index (col) #2=1 ("索引 (列)"), index (col) #3=3 ("索引 (列)"), index (col) #4=4 ("索引 (列)"), index (col) #5=5 ("索引 (列)")) -> (element #1=w1583:string[], element #2=w1582:string[], element #3=w1581:string[], element #4=w1580:string[], element #5=w1579:string[])  [unwired: 5 in]
                n1299 = call "Delete empty element from array.vi"("Array In"=w1583) -> ("Array out"=w1572:string[])  [unwired: 26 in]
                n1300 = call "Delete empty element from array.vi"("Array In"=w1579) -> ("Array out"=w1576:string[])  [unwired: 26 in]
                n1301 = call "Delete empty element from array.vi"("Array In"=w1582) -> ("Array out"=w1573:string[])  [unwired: 26 in]
                n1302 = call "Delete empty element from array.vi"("Array In"=w1581) -> ("Array out"=w1574:string[])  [unwired: 26 in]
                n1303 = call "Delete empty element from array.vi"("Array In"=w1580) -> ("Array out"=w1575:string[])  [unwired: 26 in]
                n1304 = Array Size(array=w1573) -> (size(s)=w1590:i32)
                n1305 = Array Size(array=w1575) -> (size(s)=w1593:i32)
                n1306 = Array Size(array=w1576) -> (size(s)=w1577:i32)
                n1307 = Initialize Array(37, w1590) -> (w1591:i32[])
                n1308 = Initialize Array(w1571, w1593) -> (w1592:i32[])
                n1309 = Initialize Array(w1571, w1577) -> (w1578:i32[])
                n1310 = property on="Diff Test Items" class="LstBox (严格)"("Item Names"=w1572, "Item Symbols"=i32[] [38, 37, 37, 38, 38, 37, 38, 37, 37, 37, 37, 37, 37, 37, 37, 37, 37, 37, 38, 38] ("初始化的数组")) -> ()  [unwired: 2 in, 2 out]
                n1311 = property on="Single Test Items" class="LstBox (严格)"("Item Names"=w1573, "Item Symbols"=w1591) -> ()  [unwired: 2 in, 2 out]
                n1312 = property on="S-para Pair Name" class="LstBox (严格)"("Item Names"=w1574, "Item Symbols"=i32[] [38, 38, 38, 38, 38, 38, 38, 38, 37, 37, 37, 37, 37, 37, 37, 37] ("初始化的数组")) -> ()  [unwired: 2 in, 2 out]
                n1313 = property on="NEXT Pair Name" class="LstBox (严格)"("Item Names"=w1575, "Item Symbols"=w1592) -> ()  [unwired: 2 in, 2 out]
                n1314 = property on="FEXT Pair Name" class="LstBox (严格)"("Item Names"=w1576, "Item Symbols"=w1578) -> ()  [unwired: 2 in, 2 out]
                n1315 = property on="Diff Test Items" class="LstBox (严格)"("Value"=w1567, "Top Row"=w1567) -> ()  [unwired: 2 in, 2 out]
                n1316 = property on="Single Test Items" class="LstBox (严格)"("Value"=w1567, "Top Row"=w1567) -> ()  [unwired: 2 in, 2 out]
                n1317 = property on="TDR Test Items" class="LstBox (严格)"("Value"=w1567, "Top Row"=w1567) -> ()  [unwired: 2 in, 2 out]
                n1318 = property on="NEXT Pair Name" class="LstBox (严格)"("Value"=w1567, "Top Row"=w1567) -> ()  [unwired: 2 in, 2 out]
                n1319 = property on="FEXT Pair Name" class="LstBox (严格)"("Value"=w1567, "Top Row"=w1567) -> ()  [unwired: 2 in, 2 out]
                n1320 = property on="S-para Pair Name" class="LstBox (严格)"("Value"=w1567, "Top Row"=w1567) -> ()  [unwired: 2 in, 2 out]
              }
            }
          }
          event "Default  fre": Value Change {
            n1321 = event-data() -> ()  [unwired: 1 in, 5 out]
            n1322 = case shown="\"Clear\"" "Default  fre" {
              frame "Default", Default {
                n1323 = local write "fre-save"(string[] ["2500", "4500", "5000", "5156.25", "6000", "9000", "10000", "12890", "19000", "20000"]) -> ()
              }
              frame "Clear" {
                n1324 = local write "fre-save"(string[] [] ("fre-save")) -> ()
              }
            }
          }
          event "Default": Value Change {
            n1325 = event-data() -> ()  [unwired: 1 in, 5 out]
            n1326 = case shown="真" "Default" {
              frame False {
              }
              frame True {
                n1327 = property on="Postion for \"PN&Tester&Date\" etc Fields" class="Tbl (严格)"("Value"=string[][] [["Applicant", "0", "2", "1"], ["Part Name", "0", "3", "1"], ["Part Number", "0", "4", "1"], ["Report No", "0", "2", "12"], ["Sample No", "0", "4", "12"], ["Prepared By", "0", "63", "0"], ["Approved By", "0", "63", "6"], ["Date", "0", "63", "2"], ["Thru Result", "0", "13", "5"], ["NEXT Result", "0", "45", "4"], ["FEXT Result", "0", "45", "5"]] ("Postion for \"PN&Tester&Date\" etc Fields"), "Active Cell"=T4 {"Row"=0, "Column"=0} ("编辑位置")) -> ()  [unwired: 2 in, 2 out]
              }
            }
          }
        }
      }
    }
  }
